vi "Files_Unable_to_Update.vi"(1 "error in (no error)":errorcluster, 2 "Target Path":path, 3 "Source Path":path) -> ()   [LabVIEW 2010]
uses:
  Globals/Constants_global.vi
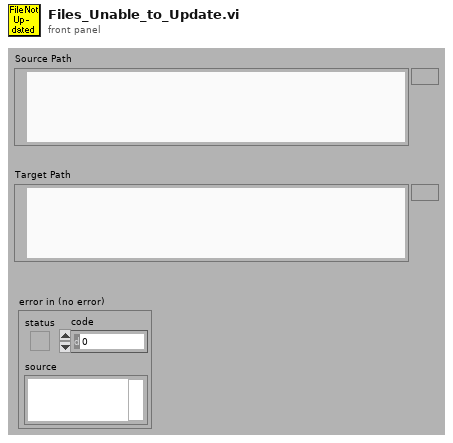
[diagram p1: front panel]
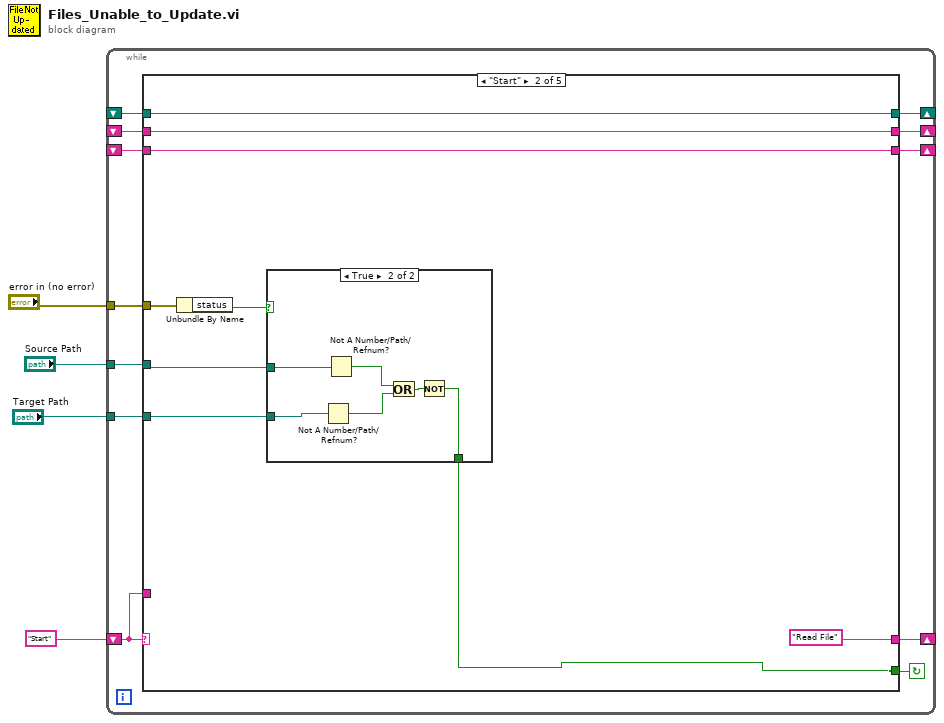
[diagram p0: block diagram]
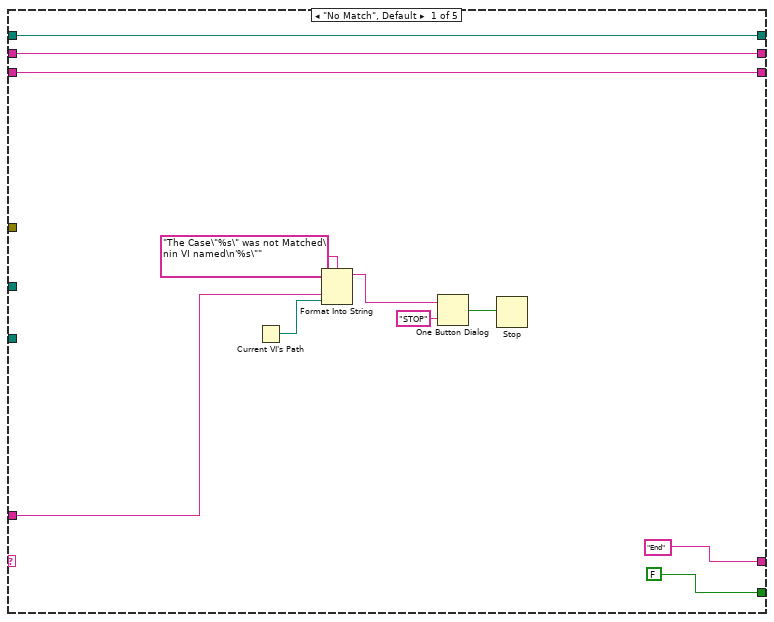
[diagram p2: hidden frame]
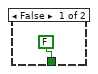
[diagram p3: hidden frame]
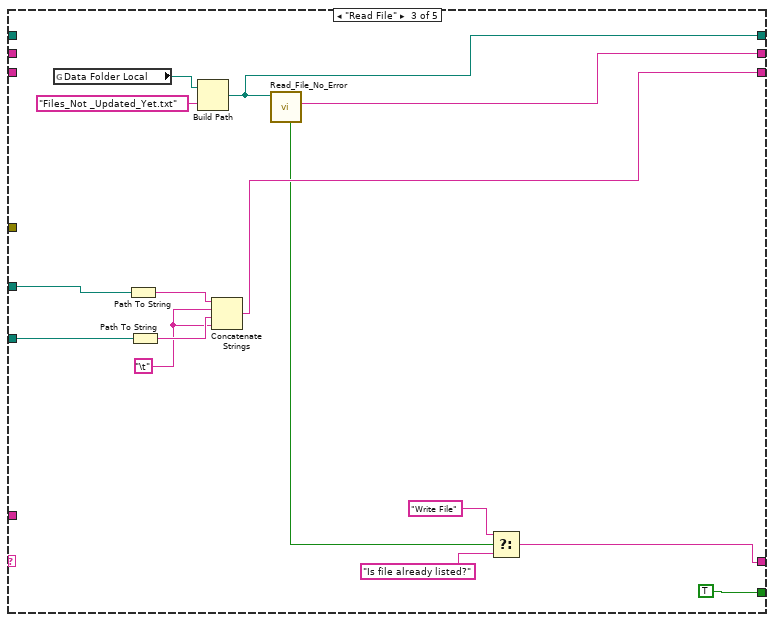
[diagram p4: hidden frame]
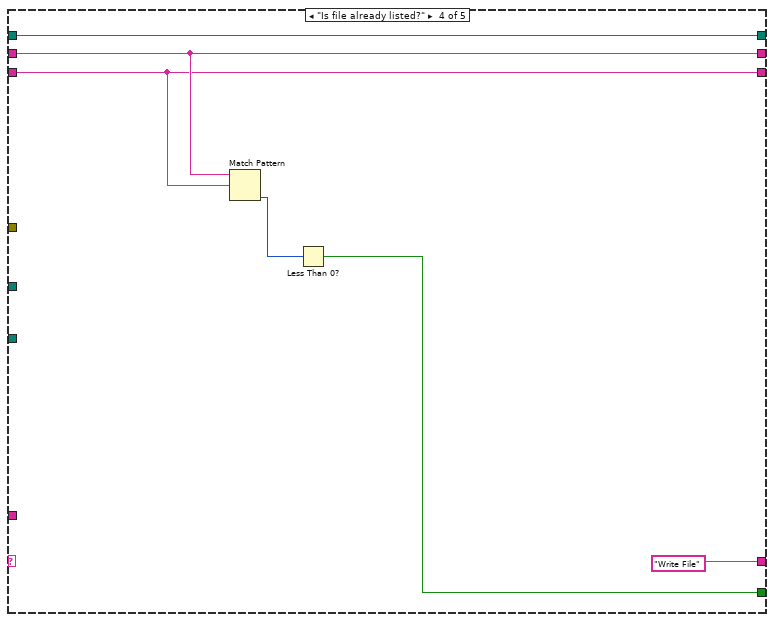
[diagram p5: hidden frame]
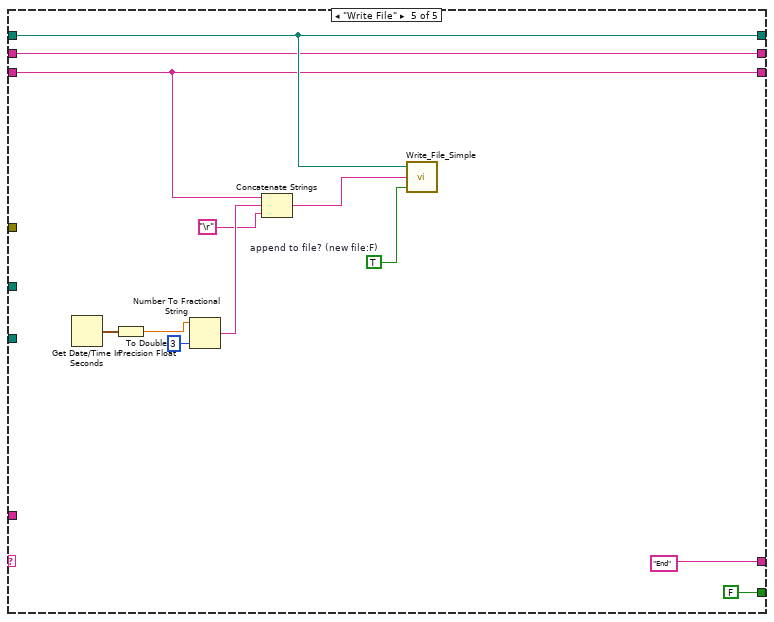
[diagram p6: hidden frame]
diagram:
  n1 = while {
    shift-left: "Start" -> [w14]
    shift-right: [w15] -> _
    tunnel: "error in (no error)" -> [w13]
    shift-right: [w12] -> _
    shift-left: _ -> [w10]
    shift-right: [w11] -> _
    shift-left: _ -> [w9]
    shift-right: [w8] -> _
    shift-left: _ -> [w7]
    tunnel: "Source Path" -> [w6]
    tunnel: "Target Path" -> [w5]
    stop <- w16 continue-if-true
    n2 = case shown="\"Start\"" w14 {
      tunnel: [FALSE w28 TRUE w62 FALSE ("status")] -> w16
      tunnel: ["End" "Read File" w46 "Write File" "End"] -> w15
      tunnel: w14 -> [w22 _ _ _ _]
      tunnel: w13 -> [_ w35 _ _ _]
      tunnel: [w19 w34 w55 w59 w75] -> w12
      tunnel: [w18 w33 w51 w61 w74] -> w11
      tunnel: w10 -> [w19 w34 _ w59 w75]
      tunnel: w9 -> [w18 w33 _ w61 w74]
      tunnel: [w17 w32 w50 w60 w70] -> w8
      tunnel: w7 -> [w17 w32 _ w60 w70]
      tunnel: w6 -> [_ w30 w45 _ _]
      tunnel: w5 -> [_ w31 w44 _ _]
      frame "No Match", Default {
        n3 = Current VI's Path() -> (path=w21:path)
        n4 = Format Into String(format string="The Case\"%s\" was not Matched\nin VI named\n'%s\"" ("Format String"), w22, w21) -> (resulting string=w25:string)  [unwired: 2 in, 1 out]
        n5 = One Button Dialog(message=w25, button name ("OK")="STOP") -> (true=w23:bool)
        n6 = Stop(stop? (T)=w23) -> ()
      }
      frame "Start" {
        n7 = Unbundle By Name(w35) -> ("status"=w29:bool)
        n8 = case shown="True" w29 {
          tunnel: w31 -> [_ w43]
          tunnel: w30 -> [_ w42]
          tunnel: [FALSE w38] -> w28
          frame False {
          }
          frame True {
            n9 = Not A Number/Path/Refnum?(number/path/refnum=w43) -> (NaN/Path/Refnum?=w41:bool)
            n10 = Not A Number/Path/Refnum?(number/path/refnum=w42) -> (NaN/Path/Refnum?=w40:bool)
            n11 = Or(x=w40, y=w41) -> (x .or. y?=w39:bool)
            n12 = Not(x=w39) -> (.not. x?=w38:bool)
          }
        }
      }
      frame "Read File" {
        w52 = "\t"
        n13 = global read "Constants_global.vi" "Data Folder Local"() -> (w57:path)
        n14 = Path To String(path=w45) -> (string=w54:string)
        n15 = Path To String(path=w44) -> (string=w53:string)
        n16 = Build Path(base path=w57, name or relative path="Files_Not _Updated_Yet.txt") -> (appended path=w55:path)
        n17 = Concatenate Strings(w54, w52, w53, w52) -> (w50:string)
        n18 = call "Read_File_No_Error.vi"("Filename"=w55) -> ("Error?"=w49:bool, "string"=w51:string)  [unwired: 2 in, 6 out]
        n19 = Select(t="Write File", s=w49, f="Is file already listed?") -> (s? t:f=w46:string)
      }
      frame "Is file already listed?" {
        n20 = Match Pattern(string=w61, regular expression=w60) -> (offset past match=w63:i32)  [unwired: 4 out]
        n21 = Less Than 0?(x=w63) -> (x < 0?=w62:bool)
      }
      frame "Write File" {
        w66 = TRUE  # append to file? (new file:F)
        n22 = Get Date/Time In Seconds() -> (seconds since 1Jan1904=w73:timestamp)
        n23 = To Double Precision Float(number=w73) -> (double precision float=w72:dbl)
        n24 = Number To Fractional String(number=w72, precision (6)=i16 3) -> (F-format string=w69:string)  [unwired: 2 out]
        n25 = Concatenate Strings(w70, w69, "\r") -> (w67:string)
        n26 = call "Write_File_Simple.vi"("append to file? (new file:F)"=w66, "character string"=w67, "file path"=w75) -> ()  [unwired: 2 out]
      }
    }
  }
